vi "Valid Name Code Point.vi"(2 "First":bool, 3 "Code Point":u32) -> (0 "Valid?":bool)   [LabVIEW 2020, in "Stream.lvlib" / "URLPattern.lvclass"]
uses:
  URLPattern.lvclass
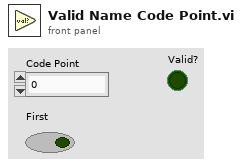
[diagram p1: front panel]
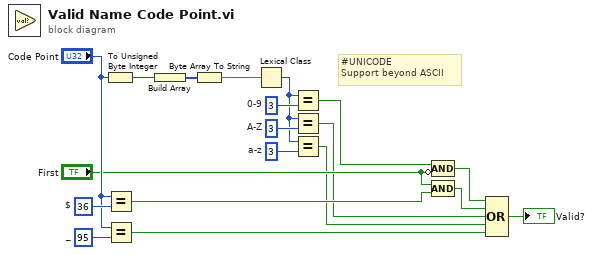
[diagram p0: block diagram]
diagram:
  w5 = i16 5  # a-z
  (unwired) i16 3 ("y")
  w6 = i16 4  # A-Z
  (unwired) i16 3 ("y")
  w15 = u32 95  # _
  w17 = u32 36  # $
  w7 = i16 3  # 0-9
  (unwired) i16 3 ("y")
  # "#UNICODE\nSupport beyond ASCII"
  n1 = To Unsigned Byte Integer(number="Code Point") -> (unsigned 8bit integer=w16:u8)
  n2 = Equal?(x="Code Point", y=w17) -> (x = y?=w11:bool)
  n3 = Equal?(x="Code Point", y=w15) -> (x = y?=w13:bool)
  n4 = Build Array(w16) -> (w19:u8[])
  n5 = Byte Array To String(unsigned byte array=w19) -> (string=w18:string)
  n6 = Lexical Class(1:w18) -> (0:w4:i16)
  n7 = Equal?(x=w4, y=w7) -> (x = y?=w1:bool)
  n8 = Equal?(x=w4, y=w6) -> (x = y?=w2:bool)
  n9 = Equal?(x=w4, y=w5) -> (x = y?=w3:bool)
  n10 = Compound Arithmetic op=AND(w1, invert "First") -> (w9:bool)
  n11 = Compound Arithmetic op=AND("First", w11) -> (w10:bool)
  n12 = Compound Arithmetic op=OR(w9, w10, w2, w3, w13) -> (→"Valid?":bool)
